vi "2D Gaussian fitting model.vi"(3 "output control":T1 caption="输出控制", 4 "data":variant caption="数据", 5 "X":dbl[](array[numeric]), 6 "a":dbl[](array[numeric])) -> (0 "error out":errorcluster caption="错误输出", 1 "f'(X,a)":dbl[][](array[numeric]), 2 "f(X,a)":dbl[](array[numeric]))   [LabVIEW 2013]
doc: "This template is the starting point for creating a model function to be passed to the Nonlinear Curve Fit.vi."
uses:
  <vilib>/gmath/NumericalOptimization/LM_output select.ctl
  <vilib>/gmath/NI_Gmath.lvlib
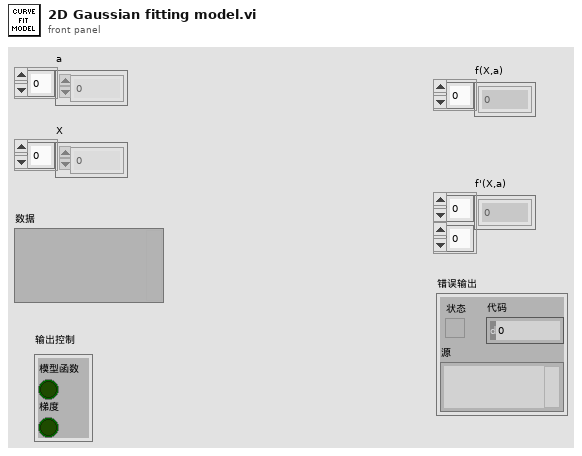
[diagram p1: front panel]
types:
  T1 = typedef "NI_Gmath.lvlib/LM_output select.ctl" = cluster{"model function":bool, "gradient":bool}
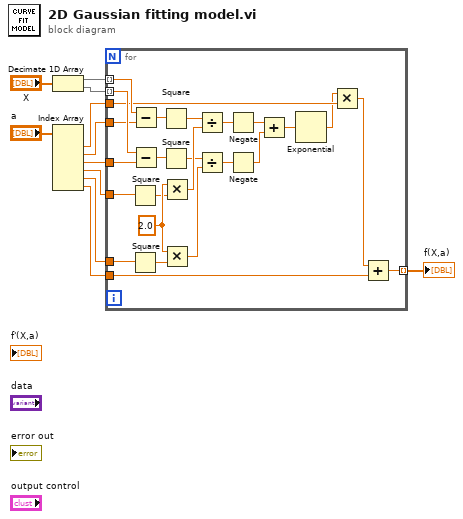
[diagram p0: block diagram]
diagram:
  n1 = Decimate 1D Array("X") -> (w3:dbl[], w2:dbl[])
  n2 = Index Array(array="a") -> (element #1=w10:dbl, element #2=w9:dbl, element #3=w8:dbl, element #4=w7:dbl, element #5=w6:dbl, element #6=w5:dbl)  [unwired: 6 in]
  n3 = for {
    tunnel: w10 -> [w16]
    tunnel: w9 -> [w34]
    tunnel: w8 -> [w35]
    tunnel: w7 -> [w28]
    tunnel: w6 -> [w29]
    tunnel: w5 -> [w13]
    tunnel: w3 -> [w33] mode=indexing
    tunnel: w2 -> [w36] mode=indexing
    tunnel: [w12] -> w1 mode=indexing
    w30 = 2.0 ("x")
    n4 = Square(x=w28) -> (x^2=w27:dbl)
    n5 = Square(x=w29) -> (x^2=w26:dbl)
    n6 = Subtract(x=w33, y=w34) -> (x-y=w32:dbl)
    n7 = Subtract(x=w36, y=w35) -> (x-y=w31:dbl)
    n8 = Square(x=w32) -> (x^2=w25:dbl)
    n9 = Square(x=w31) -> (x^2=w23:dbl)
    n10 = Multiply(x=w30, y=w27) -> (x*y=w24:dbl)
    n11 = Multiply(x=w30, y=w26) -> (x*y=w22:dbl)
    n12 = Divide(x=w25, y=w24) -> (x/y=w21:dbl)
    n13 = Divide(x=w23, y=w22) -> (x/y=w20:dbl)
    n14 = Negate(x=w21) -> (-x=w19:dbl)
    n15 = Negate(x=w20) -> (-x=w18:dbl)
    n16 = Add(x=w19, y=w18) -> (x+y=w17:dbl)
    n17 = Exponential(1:w17) -> (0:w15:dbl)
    n18 = Multiply(x=w15, y=w16) -> (x*y=w14:dbl)
    n19 = Add(x=w14, y=w13) -> (x+y=w12:dbl)
  }
  "f(X,a)" <- w1
